vi "Launch as Nested.vi"(8 "error in (no error)":errorcluster, 11 "Parent in":refnum<class "Module.lvclass">) -> (0 "error out":errorcluster, 2 "MessageQ":refnum<class "MessageQ.lvclass">, 3 "Parent":refnum<class "Module.lvclass">)   [LabVIEW 2020, in "Volatus.lvlib" / "HTTP Manager.lvclass"]
uses:
  HTTP Manager.lvclass
  HTTP Manager.lvclass/HTTP Manager.ctl
  Module/Module.lvclass
  VolatusConfig/VolatusConfigElement/VolatusConfigElement.lvclass
  C:/dev/lv20CE/relink/lv-volatus/Volatus/Module/Module.lvclass
  C:/dev/lv20CE/relink/lv-volatus/Volatus/HTTP Manager/HTTP Manager.lvclass
  MessageQ/MessageQ.lvclass
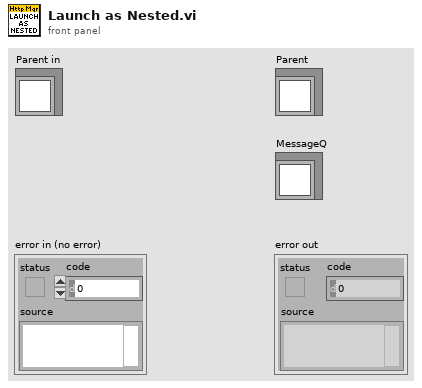
[diagram p1: front panel]
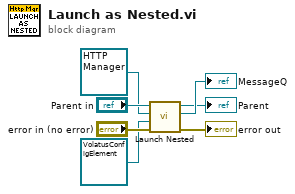
[diagram p0: block diagram]
diagram:
  n1 = call "Launch Nested.vi"("error in (no error)"="error in (no error)", "Config Element"=refnum<class "VolatusConfigElement.lvclass"> refnum, "Nested Module"=refnum<class "HTTP Manager.lvclass"> refnum ("Volatus:HTTP Manager.lvclass"), "Parent in"="Parent in") -> ("error out"=→"error out":errorcluster, "MessageQ"=→"MessageQ":refnum<class "MessageQ.lvclass">, "Parent out"=→"Parent":refnum<class "Module.lvclass">)  [unwired: 5 in]
